vi "retrieveTrajectoryData.vi"(0 "paeseHandle in":u64, 1 "path in":path=path "C:/dev/Hexagon-VTD-Custom-Device/Libraries/VC.dll", 5 "packageID":u16, 7 "playerID":u32, 9 "dataOut":u8[](array[numeric]), 11 "error in (no error)":errorcluster) -> (4 "paeseHandle out":u64, 6 "dataOut":u8[](array[numeric]), 15 "error out":errorcluster)   [LabVIEW 2023, in "RDB.lvlib"]
uses:
  RDB.lvlib
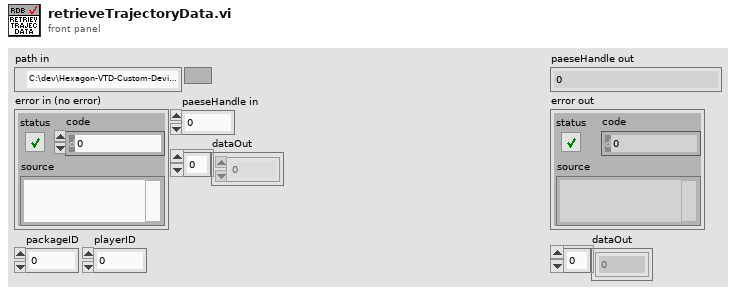
[diagram p1: front panel]
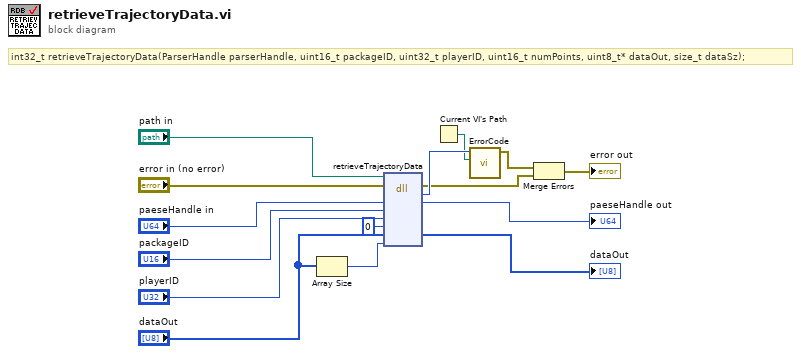
[diagram p0: block diagram]
diagram:
  # "int32_t retrieveTrajectoryData(ParserHandle parserHandle, uint16_t packageID, uint32_t playerID, uint16_t numPoints, uint8_t* dataOut, size_t dataSz);"
  n1 = Array Size(array="dataOut") -> (size(s)=w3:i32)
  n2 = dll-call lib="C:/dev/Hexagon-VTD-Custom-Device/Libraries/VC.dll" fn="retrieveTrajectoryData"(path in="path in", error in="error in (no error)", "paeseHandle"="paeseHandle in", "packageID"="packageID", "playerID"="playerID", "numPoints"=u16 0, "dataOut"="dataOut", "dataSz"=w3) -> (error out=w10:errorcluster, "return type"=w12:i32, "paeseHandle"=→"paeseHandle out":u64, "dataOut"=→"dataOut":u8[])  [unwired: 5 in, 1 out]
  n3 = Current VI's Path() -> (path=w7:path)
  n4 = call "ErrorCode.vi"("parent VI path"=w7, "return type"=w12) -> ("error out"=w11:errorcluster)  [unwired: 9 in]
  n5 = Merge Errors(w11, w10) -> (→"error out":errorcluster)
